vi "create array of lines.vi"(10 "object":T1 {"direction" step=0.1}) -> (2 "lines[]":cluster{"y":i32, "x start":i32, "x end":i32}[](array[cluster]))   [LabVIEW 2009]
uses:
  object.ctl
panel:
  out "Array":dbl[][](array[numeric])
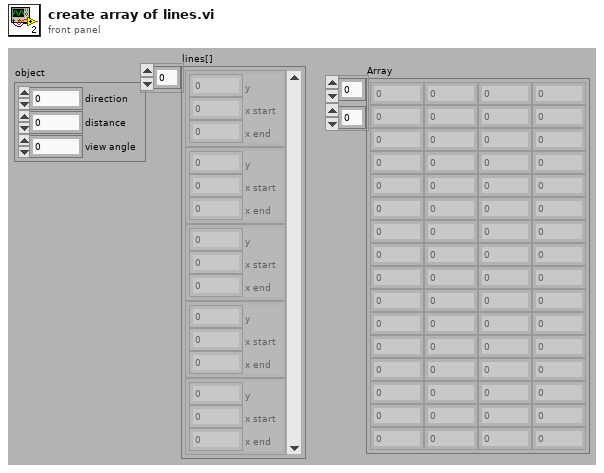
[diagram p1: front panel]
types:
  T1 = typedef "object.ctl" = cluster{"direction":dbl, "distance":u32, "view angle":dbl}
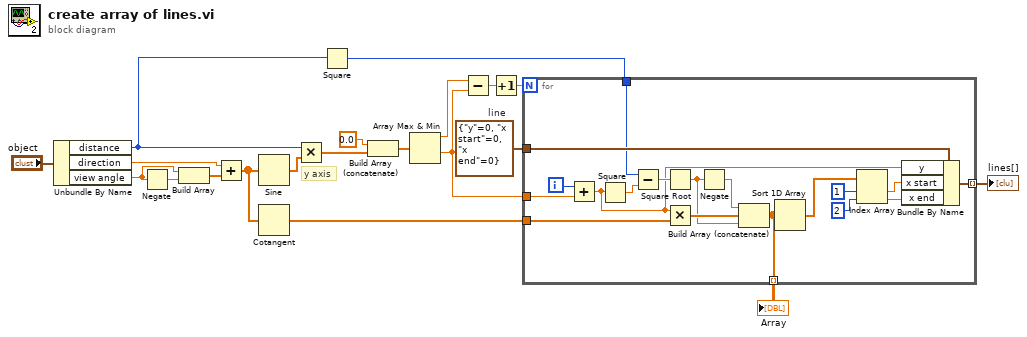
[diagram p0: block diagram]
diagram:
  w12 = cluster{"y":i32, "x start":i32, "x end":i32} {"y"=0, "x start"=0, "x end"=0}  # line
  # "y axis"
  n1 = Unbundle By Name("object") -> ("distance"=w4:u32, "direction"=w10:dbl, "view angle"=w11:dbl)
  n2 = Negate(x=w11) -> (-x=w19:dbl)
  n3 = Build Array(w11, w19) -> (w18:dbl[])
  n4 = Add(x=w10, y=w18) -> (x+y=w6:dbl[])
  n5 = Sine(x=w6) -> (sin(x)=w9:dbl[])
  n6 = Cotangent(1:w6) -> (0:w5:dbl[])
  n7 = Multiply(x=w4, y=w9) -> (x*y=w8:dbl[])
  n8 = Square(x=w4) -> (x^2=w3:u32)
  n9 = Build Array (concatenate)(0.0, w8) -> (w17:dbl[])
  n10 = Array Max & Min(array=w17) -> (max value=w15:dbl, min value=w13:dbl)  [unwired: 2 out]
  n11 = Subtract(x=w15, y=w13) -> (x-y=w7:dbl)
  n12 = Increment(x=w7) -> (x+1=w2:dbl)
  n13 = for {
    N: w2 -> [_]
    tunnel: w5 -> [w38]
    tunnel: w13 -> [w36]
    tunnel: [w35] -> w14 mode=indexing
    tunnel: w12 -> [w34]
    tunnel: w3 -> [w32]
    tunnel: [w23] -> w1 mode=indexing
    i -> [w37]
    n14 = Add(x=w37, y=w36) -> (x+y=w30:dbl)
    n15 = Square(x=w30) -> (x^2=w33:dbl)
    n16 = Subtract(x=w32, y=w33) -> (x-y=w31:dbl)
    n17 = Square Root(x=w31) -> (sqrt(x)=w22:dbl)
    n18 = Multiply(x=w30, y=w38) -> (x*y=w29:dbl[])
    n19 = Negate(x=w22) -> (-x=w21:dbl)
    n20 = Build Array (concatenate)(w21, w29, w22) -> (w23:dbl[])
    n21 = Sort 1D Array(array=w23) -> (sorted array=w28:dbl[])
    n22 = Index Array(array=w28, index #1=1 ("index"), index #2=2 ("index")) -> (element #1=w25:dbl, element #2=w24:dbl)
    n23 = Bundle By Name(cluster=w34, "y"=w30, "x start"=w25, "x end"=w24) -> (w35:cluster{"y":i32, "x start":i32, "x end":i32})
  }
  "lines[]" <- w14
  "Array" <- w1
